vi "emi_Error finder Array.vi"(5 "Error Codes":i32[](array[numeric]), 9 "error in (no error)":errorcluster) -> (6 "code":i32, 8 "In List":bool, 10 "error out":errorcluster, 13 "Is error":bool)   [LabVIEW 2010]
doc: "Find if error is one or severla error codes. Does not modify the error on the wire"
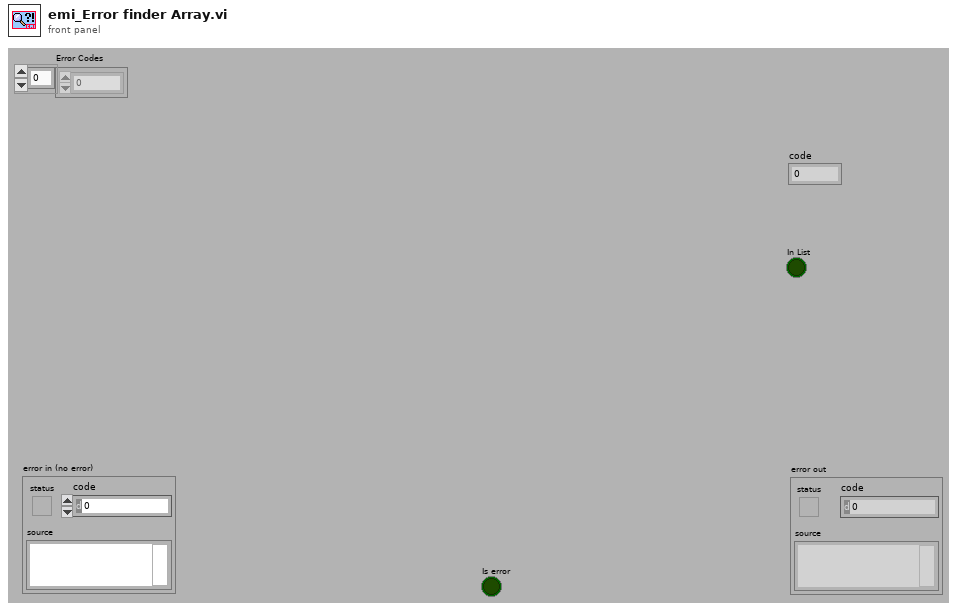
[diagram p1: front panel]
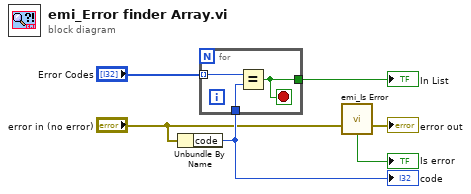
[diagram p0: block diagram]
diagram:
  n1 = Unbundle By Name("error in (no error)") -> ("code"=w5:i32)
  "code" <- w5
  n2 = for {
    tunnel: "Error Codes" -> [w9] mode=indexing
    tunnel: w5 -> [w8]
    tunnel: [w7] -> w1
    stop <- w7 stop-if-true
    n3 = Equal?(x=w9, y=w8) -> (x = y?=w7:bool)
  }
  "In List" <- w1
  n4 = call "emi_Is Error.vi"("error in (no error)"="error in (no error)") -> ("error out"=→"error out":errorcluster, "Is Error"=→"Is error":bool)  [unwired: 13 in]
